vi "Parse modbus reply.vi"(11 "read buffer":string) -> (0 "Meter reading":sgl, 1 "UnitID":i32)   [LabVIEW 2015]
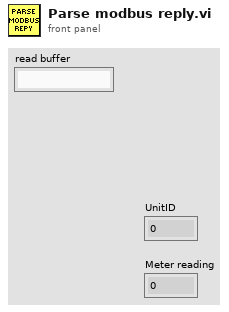
[diagram p1: front panel]
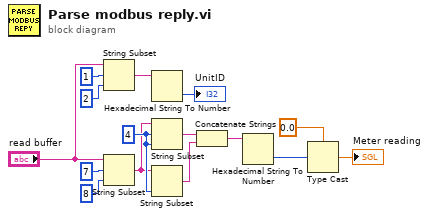
[diagram p0: block diagram]
diagram:
  w6 = 4 ("length (rest)")
  n1 = String Subset(string="read buffer", offset (0)=1, length (rest)=2 ("length (rest)")) -> (substring=w14:string)
  n2 = String Subset(string="read buffer", offset (0)=7, length (rest)=8 ("length (rest)")) -> (substring=w5:string)
  n3 = Hexadecimal String To Number(string=w14) -> (number=→"UnitID":u32)  [unwired: 2 in, 1 out]
  n4 = String Subset(string=w5, offset (0)=w6, length (rest)=w6) -> (substring=w7:string)
  n5 = String Subset(string=w5, length (rest)=w6) -> (substring=w8:string)  [unwired: 1 in]
  n6 = Concatenate Strings(w7, w8) -> (w9:string)
  n7 = Hexadecimal String To Number(string=w9) -> (number=w2:u32)  [unwired: 2 in, 1 out]
  n8 = Type Cast(type=sgl 0.0, x=w2) -> (*(type *) &x=→"Meter reading":sgl)
